vi "Delete Edge Point.vi"(0 "FSM.Graph In":refnum<class "FSM.Graph.lvclass">) -> (4 "FSM.Graph Out":refnum<class "FSM.Graph.lvclass">)   [LabVIEW 2020, in "FSM.Graph.lvclass"]
uses:
  FSM.Graph.lvclass
  FSM.Graph.lvclass/FSM.Graph.ctl
  FSM.Edge/FSM.Edge.lvclass
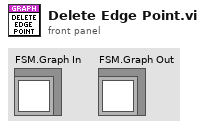
[diagram p1: front panel]
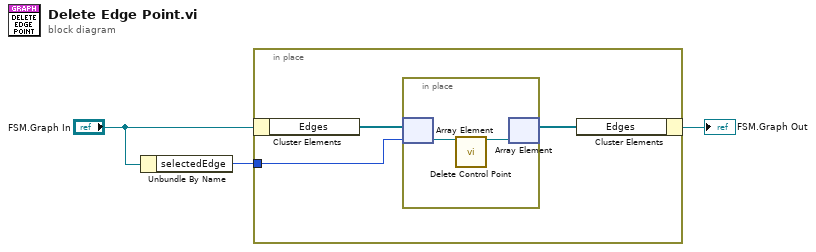
[diagram p0: block diagram]
diagram:
  n1 = Unbundle By Name("FSM.Graph In") -> ("selectedEdge"=w2:i32)
  n2 = in-place {
    in-place-border: w2 -> [w6]
    n3 = in-place-cluster #1("FSM.Graph In") -> ("Edges"=w5:refnum<class "FSM.Edge.lvclass">[])
    n4 = in-place {
      n5 = in-place-array #2(w5, w6) -> (w8:refnum<class "FSM.Edge.lvclass">)
      n6 = call "Delete Control Point.vi"("FSM.Edge In"=w8) -> ("FSM.Edge Out"=w7:refnum<class "FSM.Edge.lvclass">)  [unwired: 14 in]
      n7 = in-place-array #2(w7) -> (w4:refnum<class "FSM.Edge.lvclass">[])  [unwired: 1 out]
    }
    n8 = in-place-cluster #1("Edges"=w4) -> (→"FSM.Graph Out":refnum<class "FSM.Graph.lvclass">)
  }
